vi "Read Music Element Library.vi"(8 "error in (no error)":errorcluster, 11 "MusicElementLibrary in":refnum<class "MusicElementLibrary.lvclass">) -> (0 "error out":errorcluster, 2 "Music Element Library":refnum<class "MusicElement.lvclass">[](array[class]), 3 "MusicElementLibrary out":refnum<class "MusicElementLibrary.lvclass">)   [LabVIEW 2015, in "MusicElementLibrary.lvclass"]
uses:
  MusicElementLibrary.lvclass
  MusicElement.lvclass
  MusicElementLibrary.lvclass/MusicElementLibrary.ctl
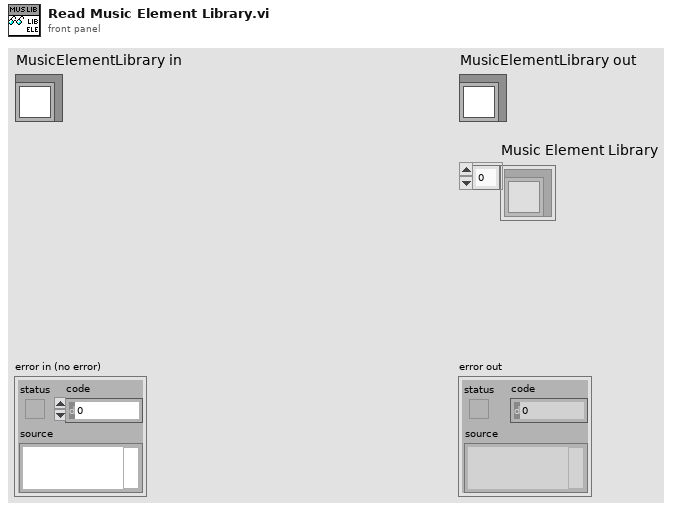
[diagram p1: front panel]
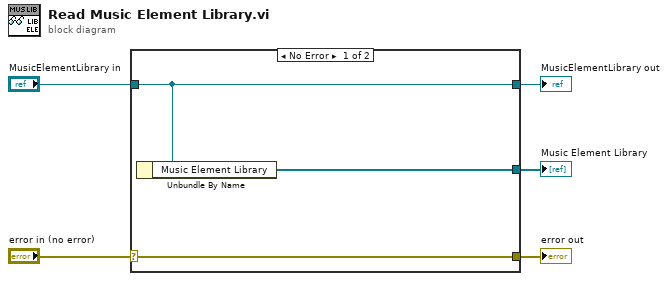
[diagram p0: block diagram]
diagram:
  n1 = case shown="No Error" "error in (no error)" {
    selector: "error in (no error)" -> [w8 w9]
    tunnel: [w8 w9] -> w4
    tunnel: [w7 w10] -> w2
    tunnel: "MusicElementLibrary in" -> [w7 w10]
    tunnel: [w6 _] -> w1
    frame No Error {
      n2 = Unbundle By Name(w7) -> ("Music Element Library"=w6:refnum<class "MusicElement.lvclass">[])
    }
    frame Error {
    }
  }
  "error out" <- w4
  "MusicElementLibrary out" <- w2
  "Music Element Library" <- w1
